vi "Memory.Pointer.Parameter Check.Size.1D.Power of 2.vi"(5 "power of 2":i16, 7 "source vi name":string, 8 "error in (no error)":errorcluster, 9 "transfer count":u64 format="%08x bytes", 10 "buffer element count":u64 format="%08x bytes", 11 "Pointer in":refnum<class "Memory.Pointer.lvclass">) -> (0 "error out":errorcluster, 1 "transfer count out":u64 format="%08x bytes", 2 "buffer element count out":u64 format="%08x bytes", 3 "Pointer out":refnum<class "Memory.Pointer.lvclass">)   [LabVIEW 2016, in "Memory.lvlib" / "Memory.Pointer.lvclass"]
uses:
  Memory.Pointer.lvclass
  Memory.Pointer.Errors.Buffer Underflow.vi
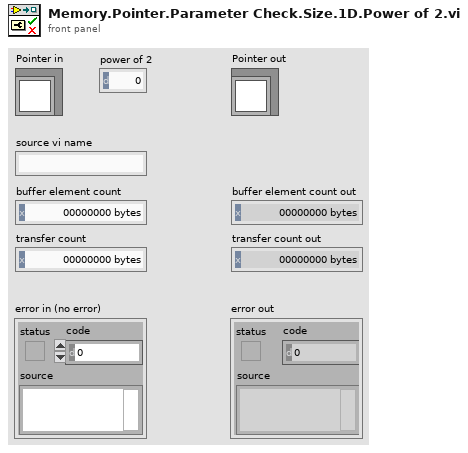
[diagram p1: front panel]
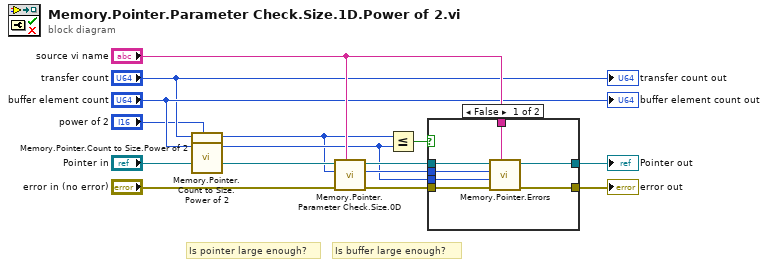
[diagram p0: block diagram]
diagram:
  # "Is buffer large enough?"
  # "Is pointer large enough?"
  n1 = call "Memory.Pointer.Count to Size.Power of 2.vi"("power of 2"="power of 2", "count"="transfer count") -> ("size"=w2:u64)  [unwired: 9 in]
  n2 = call "Memory.Pointer.Count to Size.Power of 2.vi"("power of 2"="power of 2", "count"="buffer element count") -> ("size"=w5:u64)  [unwired: 9 in]
  n3 = call "Memory.Pointer.Parameter Check.Size.0D.vi"("source vi name"="source vi name", "error in (no error)"="error in (no error)", "required size"=w2, "Pointer in"="Pointer in") -> ("error out"=w9:errorcluster, "required size out"=w7:u64, "Pointer out"=w10:refnum<class "Memory.Pointer.lvclass">)  [unwired: 5 in]
  n4 = Less Or Equal?(x=w2, y=w5) -> (x <= y?=w6:bool)
  n5 = case shown="False" w6 {
    tunnel: w10 -> [w21 w22]
    tunnel: w9 -> [w19 w23]
    tunnel: [w18 w23] -> w14
    tunnel: [w20 w22] -> w13
    tunnel: "source vi name" -> [w17 _]
    tunnel: w5 -> [w16 _]
    tunnel: w7 -> [w15 _]
    frame False {
      n6 = call-poly "Memory.Pointer.Errors.vi"("error source vi name"=w17, "error in (no error)"=w19, "actual buffer size"=w16, "required buffer size"=w15, "Pointer in"=w21) -> ("error out"=w18:errorcluster, "Pointer out"=w20:refnum<class "Memory.Pointer.lvclass">)  [unwired: 5 in]
    }
    frame True {
    }
  }
  "error out" <- w14
  "Pointer out" <- w13
  "transfer count out" <- "transfer count"
  "buffer element count out" <- "buffer element count"
